vi "Highlanders List Init.vi"(8 "error in (no error)":errorcluster, 11 "Guardian in":refnum<class "Guardian.lvclass">) -> (0 "error out":errorcluster, 3 "Guardian out":refnum<class "Guardian.lvclass">)   [LabVIEW 2026, in "TALOS.lvlib" / "Guardian.lvlib" / "Guardian.lvclass"]
uses:
  Guardian.lvclass
  Guardian.lvclass/Guardian.ctl
  TALOS.lvlib
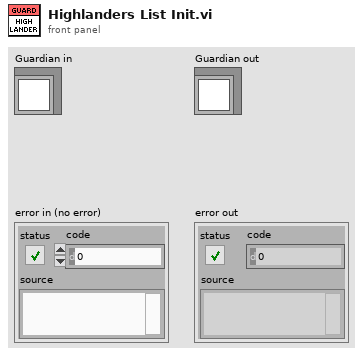
[diagram p1: front panel]
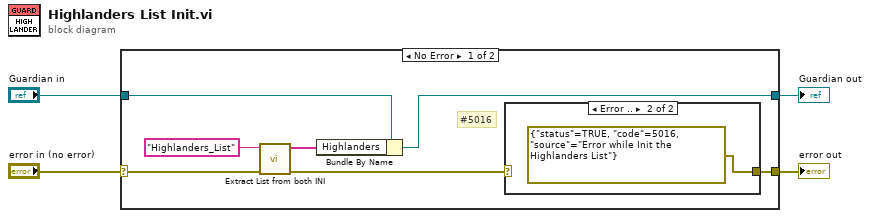
[diagram p0: block diagram]
diagram:
  n1 = case shown="No Error" "error in (no error)" {
    selector: "error in (no error)" -> [w9 w14]
    tunnel: "Guardian in" -> [w11 w15]
    tunnel: [w7 w15] -> w3
    tunnel: [w5 w14] -> w1
    frame No Error {
      # "#5016"
      n2 = call "Extract List from both INI.vi"("error in (no error)"=w9, "Parameter Name"="Highlanders_List") -> ("error out"=w6:errorcluster, "Array"=w8:string[])  [unwired: 8 in]
      n3 = Bundle By Name(cluster=w11, "Highlanders"=w8) -> (w7:refnum<class "Guardian.lvclass">)
      n4 = case shown="Error .." w6 {
        selector: w6 -> [w12 _]
        tunnel: [w12 errorcluster {"status"=TRUE, "code"=5016, "source"="Error while Init the Highlanders List"} ("error IO")] -> w5
        frame No Error {
        }
        frame Error {
        }
      }
    }
    frame Error {
    }
  }
  "Guardian out" <- w3
  "error out" <- w1
